vi "api_mqttPing.vi"(0 "mqtt.lvclass in":refnum<class "mqtt.lvclass">, 11 "error in (no error)":errorcluster) -> (4 "mqtt.lvclass out":refnum<class "mqtt.lvclass">, 6 "success":bool, 15 "error out":errorcluster)   [LabVIEW 2018, in "labview-mqtt.lvlib" / "mqtt.lvclass"]
uses:
  mqtt.lvclass
  mqttTypedef/mqttRXdataCluster.ctl
  mqttTypedef/mqttFixedHeaderResponse.ctl
  mqttTypedef/mqttQOSlevel.ctl
  mqttTypedef/mqttMessageType.ctl
  mqttCmd/mqttCmdPing/mqttCmdPing.lvclass
  D:/OneDrive/_WorkingOn/IECube/MQTT LabVIEW/mqtt-LabVIEW-master-yao/src/class/mqtt/mqttCmd/mqttCmd.lvclass
  mqttCmd/mqttCmd.lvclass/mqttCmd.ctl
  mqttCmd/mqttCmd.lvclass
  labview-mqtt.lvlib
panel:
  out "notification":T1
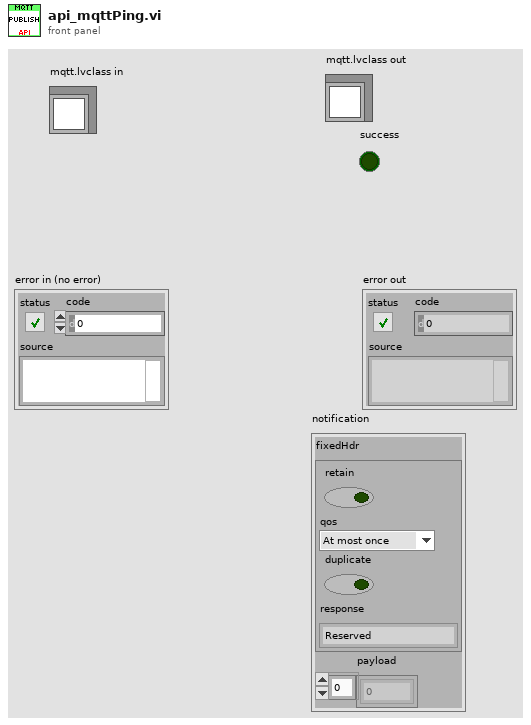
[diagram p1: front panel]
types:
  T1 = typedef "labview-mqtt.lvlib/mqttRXdataCluster.ctl" = cluster{"fixedHdr":T2, "payload":u8[]}
  T2 = typedef "labview-mqtt.lvlib/mqttFixedHeaderResponse.ctl" = cluster{"retain":bool, "qos":T3, "duplicate":bool, "response":T4}
  T3 = typedef "labview-mqtt.lvlib/mqttQOSlevel.ctl" = enum8{"At most once", "At least once", "Exactly once", "Reserved"}
  T4 = typedef "labview-mqtt.lvlib/mqttMessageType.ctl" = enum32{"Reserved", "CONNECT", "CONNACK", "PUBLISH", "PUBACK", "PUBREC", "PUBREL", "PUBCOMP", "SUBSCRIBE", "SUBACK", "UNSUBSCRIBE", "UNSUBACK", "PINGREQ", "PINGRESP", "DISCONNECT", "Reserved2"}
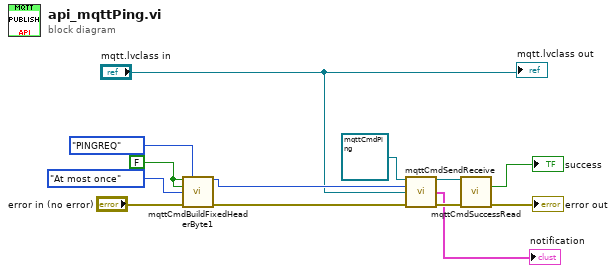
[diagram p0: block diagram]
diagram:
  w2 = FALSE ("retain(F)")
  n1 = call "mqttCmdBuildFixedHeaderByte1.vi"("retain(F)"=w2, "MessageType"=mqttMessageType."PINGREQ", "duplicate(F)"=w2, "QoS (At most once)"=mqttQOSlevel."At most once", "error in (no error)"="error in (no error)") -> ("byte1"=w3:u8, "error out"=w11:errorcluster)  [unwired: 9 in]
  n2 = call "mqttCmdSendReceive.vi"("mqttConnect in"=refnum<class "mqttCmdPing.lvclass"> refnum ("mqttCmdPing.lvclass"), "byte1"=w3, "mqtt in"="mqtt.lvclass in", "error in (no error)"=w11) -> ("mqttConnect out"=w7:refnum<class "mqttCmdPing.lvclass">, "notification"=→"notification":T1, "error out"=w6:errorcluster)  [unwired: 9 in]
  n3 = call "mqttCmdSuccessRead.vi"("mqttBrokerCommand in"=w7, "error in (no error)"=w6) -> ("success"=→"success":bool, "error out"=→"error out":errorcluster)  [unwired: 11 in, 1 out]
  "mqtt.lvclass out" <- "mqtt.lvclass in"
